vi "getCrossCoordinates.vi"(11 "Grid":T1) -> (2 "verticalCoor":cluster{dbl, dbl}, 3 "horizontalCoor":cluster{dbl, dbl})   [LabVIEW 2020]
uses:
  <vilib>/imath/engines/lvmath2/RunTimeEngine/NodeEndStatement/NIMS_NodeEndStatement_Output.vi
  <instcachedir>/0/NIMS_NodeEndStatement_Output_53EC0D466D134D7ABD903AC30B43404B.lvgen/NIMS_NodeEndStatement_Output_53EC0D466D134D7ABD903AC30B43404B_000.vi
  <vilib>/imath/engines/lvmath2/RunTimeEngine/ErrorHandling/NIMS_Finalize Error.vi
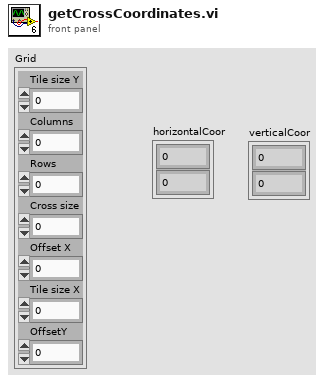
[diagram p1: front panel]
types:
  T1 = cluster{"Tile size Y":dbl, "Columns":dbl, "Rows":dbl, "Cross size":dbl, "Offset X":dbl, "Tile size X":dbl, "OffsetY":dbl}
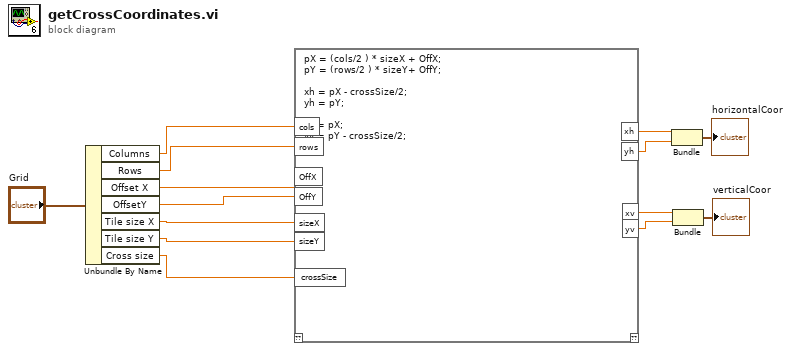
[diagram p0: block diagram]
diagram:
  n1 = Unbundle By Name("Grid") -> ("Columns"=w11:dbl, "Rows"=w10:dbl, "Offset X"=w9:dbl, "OffsetY"=w8:dbl, "Tile size X"=w7:dbl, "Tile size Y"=w6:dbl, "Cross size"=w5:dbl)
  n2 = mathscript code="pX = (cols/2 ) * sizeX + OffX;\npY = (rows/2 ) * sizeY+ OffY;\n\nxh = pX - crossSize/2;\nyh = pY;\n\nxv = pX;\nyv = pY - crossSize/2;"("cols"=w11, "rows"=w10, "OffX"=w9, "OffY"=w8, "sizeX"=w7, "sizeY"=w6, "crossSize"=w5) -> ("xh"=w4:dbl, "yh"=w3:dbl, "xv"=w2:dbl, "yv"=w1:dbl)  [unwired: 1 in, 1 out]
  n3 = Bundle("xh"=w4, "yh"=w3) -> (→"horizontalCoor":cluster{"xh":dbl, "yh":dbl})  [unwired: 1 in]
  n4 = Bundle("xv"=w2, "yv"=w1) -> (→"verticalCoor":cluster{"xv":dbl, "yv":dbl})  [unwired: 1 in]
